vi "Menu_Property Node.vi"(11 "Affected Items Out":T1) -> (3 "Menu Items To Add":T2(array[cluster]))   [LabVIEW 2023]
uses:
  top/BundleMagic.ctl
  controls/action enum.ctl
panel:
  out "element":refnum<vi>
  out "Enabled Status":enum8{"Enabled", "Disabled"}[](array[ring])
  out "Menu Item Display Name":string[](array[string])
  out "Position In Menu":T3(array[cluster])
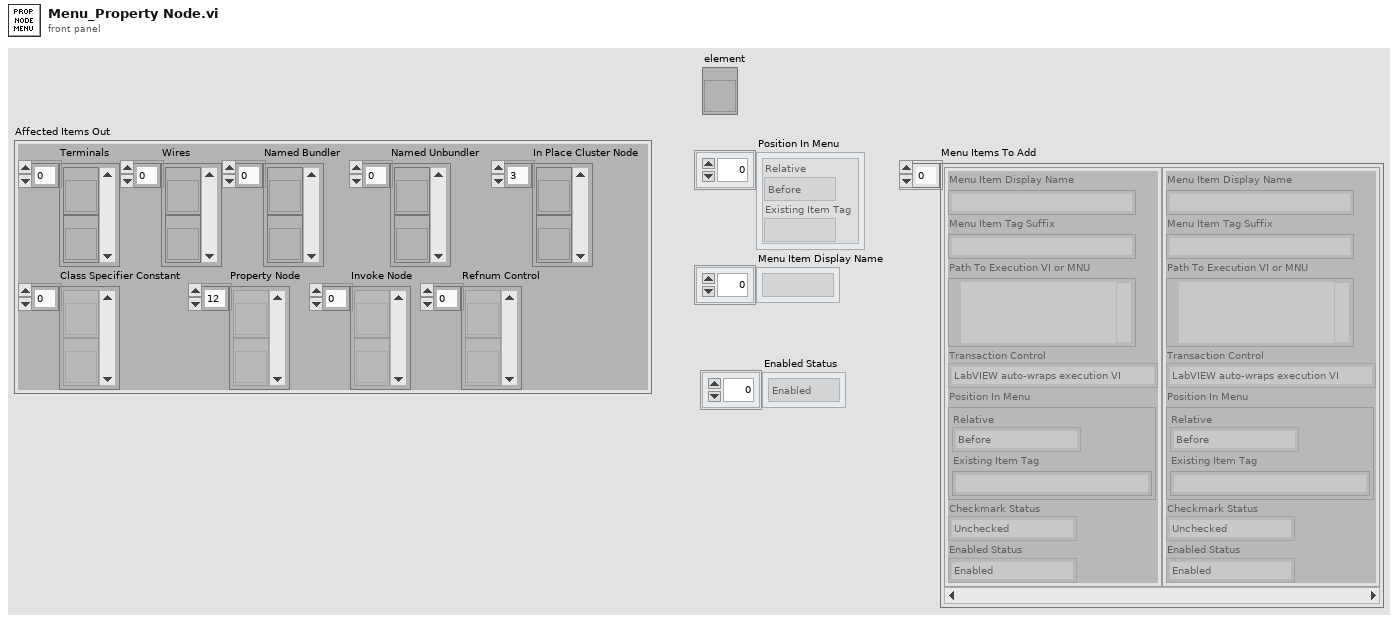
[diagram p1: front panel]
types:
  T1 = typedef "BundleMagic.ctl" = cluster{"Terminals":refnum<vi>[], "Wires":refnum<vi>[], "Named Bundler":refnum<vi>[], "Named Unbundler":refnum<vi>[], "In Place Cluster Node":refnum<vi>[], "Class Specifier Constant":refnum<vi>[], "Property Node":refnum<vi>[], "Invoke Node":refnum<vi>[], "Refnum Control":refnum<vi>[]}
  T2 = cluster{"Menu Item Display Name":string, "Menu Item Tag Suffix":string, "Path To Execution VI or MNU":path, "Transaction Control":enum8{"LabVIEW auto-wraps execution VI", "Execution VI will define if needed"}, "Position In Menu":cluster{"Relative":enum8{"Before", "Instead of", "After", "Into Submenu"}, "Existing Item Tag":string}, "Checkmark Status":enum8{"Unchecked", "Checked"}, "Enabled Status":enum8{"Enabled", "Disabled"}}[]
  T3 = cluster{"Relative":enum8{"Before", "Instead of", "After", "Into Submenu"}, "Existing Item Tag":string}[]
  T4 = typedef "action enum.ctl" = enum16{"[NONE]", "APP_SEPARATOR", "Wire Bundle", "Wire Unbundle", "Terminal Unbundle", "Terminal Bundle", "Bundler Move Up", "Bundler Move Down", "Bundler Insert", "Bundler Remove", "Bundler Remove Unwired", "Bundler Rearrange", "In Place Insert", "In Place Remove", "In Place Remove Unwired", "In Place Rearrange", "Wire Properties", "Wire Method", "Terminal Properties", "Terminal Method", "Property Move Up", "Property Move Down", "Properties Insert", "Properties Remove", "Properties Remove Unwired", "Properties Rearrange", "Method Change", "Class For Constant", "Class For Control", "Class For Node", "Class Name to Clipboard"}
  T5 = cluster{"Menu Item Display Name":string, "Menu Item Tag Suffix":string, "Path To Execution VI or MNU":path, "Transaction Control":enum8{"LabVIEW auto-wraps execution VI", "Execution VI will define if needed"}, "Position In Menu":cluster{"Relative":enum8{"Before", "Instead of", "After", "Into Submenu"}, "Existing Item Tag":string}, "Checkmark Status":enum8{"Unchecked", "Checked"}, "Enabled Status":enum8{"Enabled", "Disabled"}}
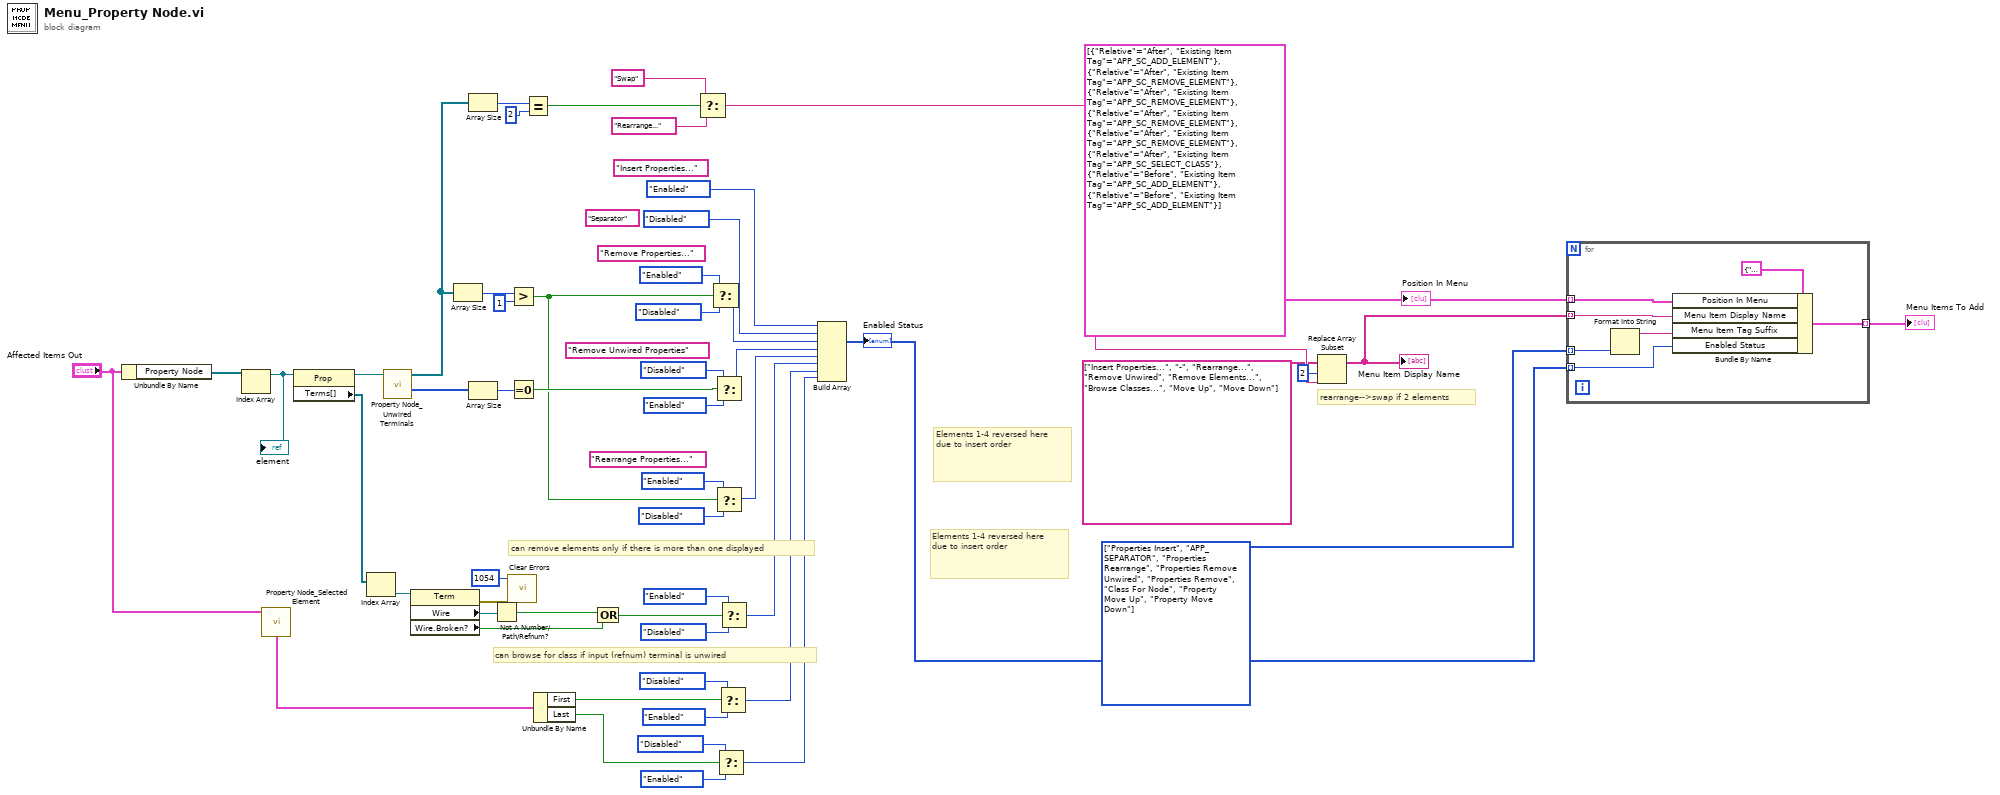
[diagram p0: block diagram]
diagram:
  (unwired) "Separator" ("Menu Item Display Name")
  (unwired) "Rearrange Properties..." ("Menu Item Display Name")
  (unwired) "Remove Unwired Properties" ("Menu Item Display Name")
  (unwired) "Remove Properties..." ("Menu Item Display Name")
  (unwired) "Insert Properties..." ("Menu Item Display Name")
  w55 = T3 [{"Relative"=enum."After", "Existing Item Tag"="APP_SC_ADD_ELEMENT"}, {"Relative"=enum."After", "Existing Item Tag"="APP_SC_REMOVE_ELEMENT"}, {"Relative"=enum."After", "Existing Item Tag"="APP_SC_REMOVE_ELEMENT"}, {"Relative"=enum."After", "Existing Item Tag"="APP_SC_REMOVE_ELEMENT"}, {"Relative"=enum."After", "Existing Item Tag"="APP_SC_REMOVE_ELEMENT"}, {"Relative"=enum."After", "Existing Item Tag"="APP_SC_SELECT_CLASS"}, {"Relative"=enum."Before", "Existing Item Tag"="APP_SC_ADD_ELEMENT"}, {"Relative"=enum."Before", "Existing Item Tag"="APP_SC_ADD_ELEMENT"}]
  w54 = T4[] [enum."Properties Insert", enum."APP_SEPARATOR", enum."Properties Rearrange", enum."Properties Remove Unwired", enum."Properties Remove", enum."Class For Node", enum."Property Move Up", enum."Property Move Down"] items=["[NONE]", "APP_SEPARATOR", "Wire Bundle", "Wire Unbundle", "Terminal Unbundle", "Terminal Bundle", "Bundler Move Up", "Bundler Move Down", "Bundler Insert", "Bundler Remove", "Bundler Remove Unwired", "Bundler Rearrange", "In Place Insert", "In Place Remove", "In Place Remove Unwired", "In Place Rearrange", "Wire Properties", "Wire Method", "Terminal Properties", "Terminal Method", "Property Move Up", "Property Move Down", "Properties Insert", "Properties Remove", "Properties Remove Unwired", "Properties Rearrange", "Method Change", "Class For Constant", "Class For Control", "Class For Node", "Class Name to Clipboard"]
  # "rearrange-->swap if 2 elements"
  # "can remove elements only if there is more than one displayed"
  # "can browse for class if input (refnum) terminal is unwired"
  # "Elements 1-4 reversed here due to insert order"
  # "Elements 1-4 reversed here due to insert order"
  n1 = Unbundle By Name("Affected Items Out") -> ("Property Node"=w52:refnum<vi>[])
  n2 = Index Array(array=w52) -> (element=w22:refnum<vi>)  [unwired: 1 in]
  "element" <- w22
  n3 = call "Property Node_Selected Element.vi"("Affected Items"="Affected Items Out") -> ("Element details"=w20:cluster{"First":bool, "Last":bool})  [unwired: 5 in, 5 out]
  n4 = property class="Prop"(reference=w22) -> (reference out=w41:refnum<vi>, "Terms[]"=w49:refnum<vi>[])  [unwired: 1 in, 1 out]
  n5 = Index Array(array=w49) -> (element=w48:refnum<vi>)  [unwired: 1 in]
  n6 = call "Property Node_Unwired Terminals.vi"("Property Node Ref"=w41) -> ("Unwired Indices For Removal"=w33:i32[], "Property Items[]"=w8:refnum<vi>[])  [unwired: 7 in, 2 out]
  n7 = property class="Term"(reference=w48) -> (error out=w29:errorcluster, "Wire"=w47:refnum<vi>, "Wire.Broken?"=w32:bool)  [unwired: 1 in, 1 out]
  n8 = Array Size(array=w8) -> (size(s)=w51:i32)
  n9 = Array Size(array=w8) -> (size(s)=w10:i32)
  n10 = Array Size(array=w33) -> (size(s)=w39:i32)
  n11 = Not A Number/Path/Refnum?(number/path/refnum=w47) -> (NaN/Path/Refnum?=w31:bool)
  n12 = call <vilib>:"Clear Errors.vi"("error in (no error)"=w29, "specific error code to clear (0: all)"=1054) -> ()  [unwired: 4 in, 2 out]
  n13 = Greater?(x=w51, y=1) -> (0:w23:bool)
  n14 = Equal To 0?(x=w39) -> (x = 0?=w38:bool)
  n15 = Equal?(x=w10, y=2) -> (x = y?=w9:bool)
  n16 = Unbundle By Name(w20) -> ("First"=w15:bool, "Last"=w14:bool)
  n17 = Compound Arithmetic op=OR(w31, w32) -> (w30:bool)
  n18 = Select(t="Swap" ("Menu Item Display Name"), s=w9, f="Rearrange..." ("Menu Item Display Name")) -> (s? t:f=w4:string)
  n19 = Select(t=enum8{"Enabled", "Disabled"}."Enabled" ("Enabled Status"), s=w23, f=enum8{"Enabled", "Disabled"}."Disabled" ("Enabled Status")) -> (s? t:f=w24:enum8{"Enabled", "Disabled"})
  n20 = Select(t=enum8{"Enabled", "Disabled"}."Disabled" ("Enabled Status"), s=w38, f=enum8{"Enabled", "Disabled"}."Enabled" ("Enabled Status")) -> (s? t:f=w35:enum8{"Enabled", "Disabled"})
  n21 = Select(t=enum8{"Enabled", "Disabled"}."Enabled" ("Enabled Status"), s=w23, f=enum8{"Enabled", "Disabled"}."Disabled" ("Enabled Status")) -> (s? t:f=w40:enum8{"Enabled", "Disabled"})
  n22 = Select(t=enum8{"Enabled", "Disabled"}."Disabled" ("Enabled Status"), s=w14, f=enum8{"Enabled", "Disabled"}."Enabled" ("Enabled Status")) -> (s? t:f=w12:enum8{"Enabled", "Disabled"})
  n23 = Select(t=enum8{"Enabled", "Disabled"}."Disabled" ("Enabled Status"), s=w15, f=enum8{"Enabled", "Disabled"}."Enabled" ("Enabled Status")) -> (s? t:f=w13:enum8{"Enabled", "Disabled"})
  n24 = Select(t=enum8{"Enabled", "Disabled"}."Enabled" ("Enabled Status"), s=w30, f=enum8{"Enabled", "Disabled"}."Disabled" ("Enabled Status")) -> (s? t:f=w42:enum8{"Enabled", "Disabled"})
  n25 = Build Array(enum8{"Enabled", "Disabled"}."Enabled" ("Enabled Status"), enum8{"Enabled", "Disabled"}."Disabled" ("Enabled Status"), w24, w35, w40, w42, w13, w12) -> (w34:enum8{"Enabled", "Disabled"}[])
  "Enabled Status" <- w34
  n26 = Replace Array Subset(array=string[] ["Insert Properties...", "-", "Rearrange...", "Remove Unwired", "Remove Elements...", "Browse Classes...", "Move Up", "Move Down"], new element=w4, index=2) -> (w2:string[])
  "Menu Item Display Name" <- w2
  n27 = for {
    tunnel: [w62] -> w53 mode=indexing
    tunnel: w2 -> [w61] mode=indexing
    tunnel: w54 -> [w56] mode=indexing
    tunnel: w55 -> [w59] mode=indexing
    tunnel: w34 -> [w58] mode=indexing
    n28 = Format Into String(w56) -> (resulting string=w57:string)  [unwired: 3 in, 1 out]
    n29 = Bundle By Name(cluster=T5 {"Menu Item Display Name"="", "Menu Item Tag Suffix"="", "Path To Execution VI or MNU"=path "", "Transaction Control"=enum."LabVIEW auto-wraps execution VI", "Position In Menu"={"Relative"=enum."Before", "Existing Item Tag"=""}, "Checkmark Status"=enum."Unchecked", "Enabled Status"=enum."Enabled"} ("Cluster"), "Position In Menu"=w59, "Menu Item Display Name"=w61, "Menu Item Tag Suffix"=w57, "Enabled Status"=w58) -> (w62:T5)
  }
  "Menu Items To Add" <- w53
  "Position In Menu" <- w55
